vi "Run Nested Actor and add ActorRef Queue Ref.vi"(8 "error in (no error)":errorcluster, 10 "Nested Module":refnum<class "ModuleAbstract.lvclass">, 11 "LaunchingModule In":refnum<class "ModuleAbstract.lvclass">) -> (0 "error out":errorcluster, 2 "Nested Actor's Enqueuer":refnum<class "Message Enqueuer.lvclass">, 3 "LaunchingModule Out":refnum<class "ModuleAbstract.lvclass">)   [LabVIEW 2019, in "ModuleAbstract.lvlib" / "ModuleAbstract.lvclass"]
uses:
  ModuleAbstract.lvclass
  C:/Program Files (x86)/National Instruments/LabVIEW 2019/vi.lib/ActorFramework/Actor/Actor.lvclass
  <vilib>/ActorFramework/Message Enqueuer/Message Enqueuer.lvclass
  ModuleAbstract.lvclass/ModuleAbstract.ctl
  Containers/ActorRefContainer/ActorRefContainer.lvclass
  <vilib>/ActorFramework/Actor/Actor.lvclass
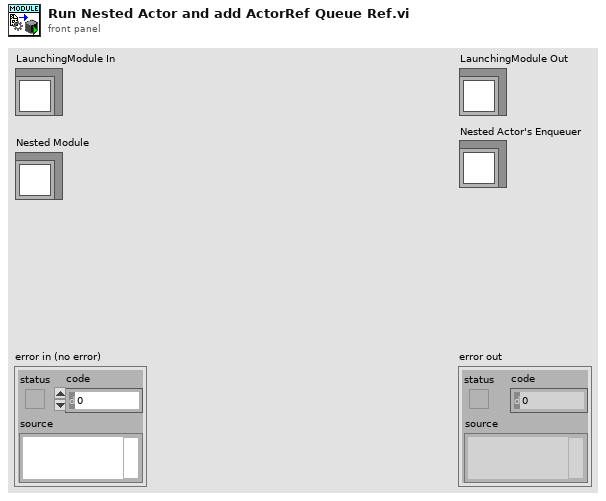
[diagram p1: front panel]
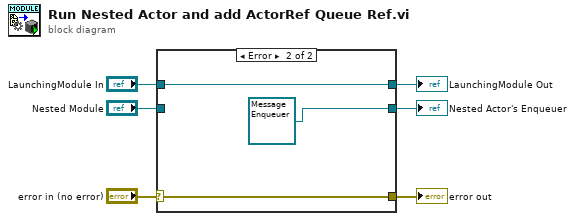
[diagram p0: block diagram]
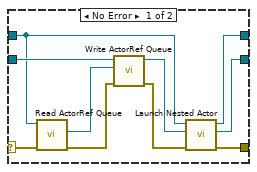
[diagram p2: hidden frame]
diagram:
  n1 = case shown="Error" "error in (no error)" {
    selector: "error in (no error)" -> [w14 w19]
    tunnel: [w11 w19] -> w5
    tunnel: [w7 refnum<class "Message Enqueuer.lvclass"> refnum ("Actor Framework:Message Enqueuer")] -> w1
    tunnel: "Nested Module" -> [w16 _]
    tunnel: "LaunchingModule In" -> [w9 w18]
    tunnel: [w8 w18] -> w2
    frame No Error {
      n2 = call "Read ActorRef Queue.vi"("error in (no error)"=w14, "ModuleAbstract in"=w9) -> ("error out"=w13:errorcluster, "ActorRef Queue"=w15:refnum<queue>)  [unwired: 7 in, 1 out]
      n3 = call "Write ActorRef Queue.vi"("error in (no error)"=w13, "ActorRef Queue"=w15, "ModuleAbstract in"=w16) -> ("error out"=w12:errorcluster, "ModuleAbstract out"=w10:refnum<class "ModuleAbstract.lvclass">)  [unwired: 7 in]
      n4 = call <vilib>:"Launch Nested Actor.vi"("error in (no error)"=w12, "Nested Actor"=w10, "Caller Actor in"=w9) -> ("error out"=w11:errorcluster, "Nested Actor's Enqueuer"=w7:refnum<class "Message Enqueuer.lvclass">, "Caller Actor out"=w8:refnum<class "ModuleAbstract.lvclass">)  [unwired: 6 in]
    }
    frame Error {
    }
  }
  "error out" <- w5
  "LaunchingModule Out" <- w2
  "Nested Actor's Enqueuer" <- w1
